vi "Assign Timing.vi"(8 "error in (no error)":errorcluster, 11 "Master Slave in":refnum<class "Master Slave.lvclass">) -> (0 "error out":errorcluster, 3 "Master Slave out":refnum<class "Master Slave.lvclass">)   [LabVIEW 2018, in "Data Acquisition.lvlib" / "Master Slave.lvclass"]
uses:
  Master Slave.lvclass
  C:/Users/Jeff Tipps/Documents/DAQMan/source/Classes/Data Acquisition/Class Chassis Tasks/Chassis Tasks.lvclass
  Class Chassis Tasks/Chassis Tasks.lvclass/Chassis Tasks.ctl
  Class Chassis Tasks/Read HS DAQ Task.vi
  Class Chassis Tasks/Read LS DAQ Task.vi
  Class Chassis Tasks/Write HS DAQ Task.vi
  Class Chassis Tasks/Write LS DAQ Task.vi
  Class Chassis Tasks/Chassis Tasks.lvclass
  Class DAQ Task/DAQ Task.lvclass
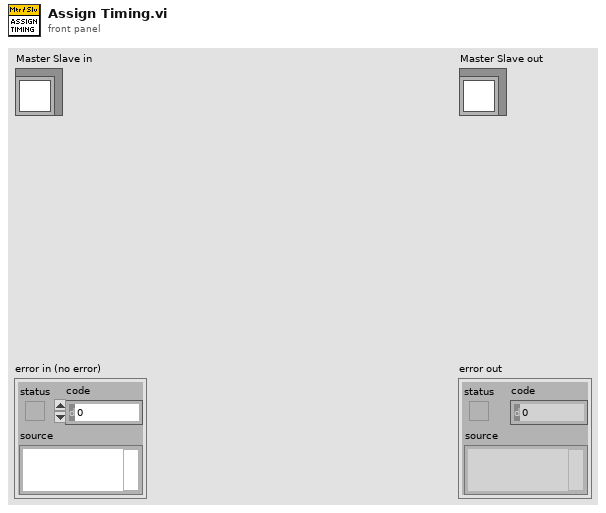
[diagram p1: front panel]
types:
  T1 = typedef "Data Acquisition.lvlib/DAQ Task.lvclass/Master Timing Info.ctl" = cluster{"SampClk.Timebase.Src":tag, "SampClk.Timebase.Rate":dbl, "Start.Term":tag}
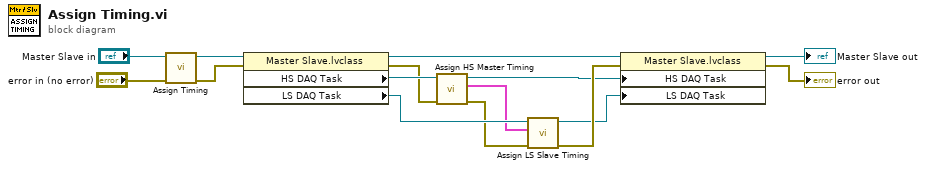
[diagram p0: block diagram]
diagram:
  n1 = call-parent "Assign Timing.vi"("error in (no error)"="error in (no error)", "Chassis Tasks in"="Master Slave in") -> ("error out"=w2:errorcluster, "Chassis Tasks out"=w3:refnum<class "Master Slave.lvclass">)  [unwired: 8 in]
  n2 = property class="Master Slave.lvclass"(reference=w3, error in=w2) -> (reference out=w14:refnum<class "Master Slave.lvclass">, error out=w9:errorcluster, "HS DAQ Task"=w11:refnum<class "DAQ Task.lvclass">, "LS DAQ Task"=w8:refnum<class "DAQ Task.lvclass">)
  n3 = call "Assign HS Master Timing.vi"("error in (no error)"=w9, "DAQ Task in"=w11) -> ("error out"=w7:errorcluster, "MasterTimingInfo"=w5:T1, "DAQ Task out"=w10:refnum<class "DAQ Task.lvclass">)  [unwired: 7 in]
  n4 = call "Assign LS Slave Timing.vi"("error in (no error)"=w7, "MasterTimingInfo"=w5, "DAQ Task in"=w8) -> ("error out"=w15:errorcluster, "DAQ Task out"=w6:refnum<class "DAQ Task.lvclass">)  [unwired: 7 in]
  n5 = property class="Master Slave.lvclass"(reference=w14, error in=w15, "HS DAQ Task"=w10, "LS DAQ Task"=w6) -> (reference out=→"Master Slave out":refnum<class "Master Slave.lvclass">, error out=→"error out":errorcluster)
